vi "Run Action_Do.vi"(8 "error in (no error)":errorcluster, 11 "Build Named Build Specification":refnum<class "Build Named Build Specification.lvclass">) -> (0 "error out":errorcluster, 1 "Success?":bool, 3 "Report Array":refnum<class "Report Data.lvclass">[](array[class]))   [LabVIEW 2020, in "ProjectBuilder.lvlib" / "Build Named Build Specification.lvclass"]
uses:
  Build Named Build Specification.lvclass
  C:/Current projects/WS/LV32.2020..ProjectBuilder/Class/Action/Project Action/Project Action.lvclass
  Data/Report Data/Report Data.lvclass
  Action/Project Action/Project Action.lvclass/Project Action.ctl
  Build Named Build Specification.lvclass/Build Named Build Specification.ctl
  Build Named Build Specification Data/Build Named Build Specification Data.lvclass/Build Named Build Specification Data.ctl
  Build Named Build Specification Data/Build Named Build Specification Data.lvclass
  C:/Current projects/WS/LV32.2020..ProjectBuilder/Class/Data/Report Data/Report Data.lvclass
  <vilib>/AppBuilder/AB_API_Simple/Build (path).vi
  <vilib>/AppBuilder/AB_API_Simple/NI_App_Builder_API.lvlib
  Action/Project Action/Project Action.lvclass
  C:/Current projects/WS/LV32.2020..ProjectBuilder/Interface/Project Action Interface/Project Action Interface.lvclass
  C:/Current projects/WS/LV32.2020..ProjectBuilder/Class/Build Named Build Specification/Build Named Build Specification.lvclass
  C:/Current projects/WS/LV32.2020..ProjectBuilder/Class/Build Named Build Specification/Build Named Build Specification Data/Build Named Build Specification Data.lvclass
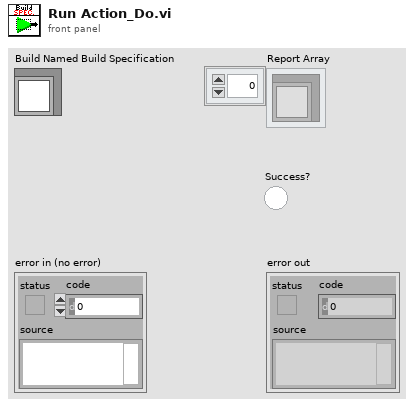
[diagram p1: front panel]
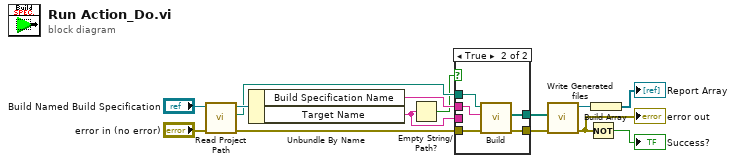
[diagram p0: block diagram]
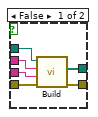
[diagram p2: hidden frame]
diagram:
  n1 = call "Read Project Path.vi"("error in (no error)"="error in (no error)", "Project Action in"="Build Named Build Specification") -> ("error out"=w9:errorcluster, "Project Path"=w11:path, "Project Action out"=w12:refnum<class "Build Named Build Specification.lvclass">)  [unwired: 7 in]
  n2 = Unbundle By Name(w12) -> ("Build Specification Name"=w10:string, "Target Name"=w1:string)
  n3 = Empty String/Path?(string/path=w1) -> (empty?=w2:bool)
  n4 = case shown="True" w2 {
    tunnel: w11 -> [w20 w25]
    tunnel: w10 -> [w19 w24]
    tunnel: w1 -> [w18 _]
    tunnel: w9 -> [w17 w23]
    tunnel: [w16 w22] -> w7
    tunnel: [w15 w21] -> w5
    frame False {
      n5 = call-poly <vilib>:"Build.vi"("error in (no error)"=w17, "Name of target (My Computer)"=w18, "Name of build specification (if empty: build all)"=w19, "Path to project"=w20) -> ("error out"=w16:errorcluster, "Generated files"=w15:path[])  [unwired: 6 in]
    }
    frame True {
      n6 = call-poly <vilib>:"Build.vi"("error in (no error)"=w23, "Name of build specification (if empty: build all)"=w24, "Path to project"=w25) -> ("error out"=w22:errorcluster, "Generated files"=w21:path[])  [unwired: 7 in]
    }
  }
  n7 = call "Write Generated files.vi"("error in (no error)"=w7, "Generated files"=w5) -> ("error out"=w6:errorcluster, "Build Named Build Specification Data out"=w4:refnum<class "Build Named Build Specification Data.lvclass">)  [unwired: 8 in]
  "error out" <- w6
  n8 = Not(x=w6) -> (.not. x?=→"Success?":bool)
  n9 = Build Array(w4) -> (→"Report Array":refnum<class "Build Named Build Specification Data.lvclass">[])
